vi "SocketQueue.vi"() -> (3 "SocketQueue":T1)   [LabVIEW 2018]
uses:
  SocketQueue.ctl
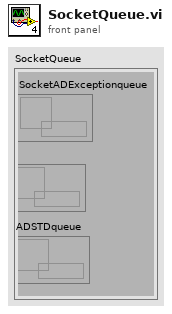
[diagram p1: front panel]
types:
  T1 = typedef "SocketQueue.ctl" = cluster{"ADSTDqueue ":refnum<queue>, "SocketADExceptionqueue":refnum<queue>, "  SocketAD":refnum<queue>}
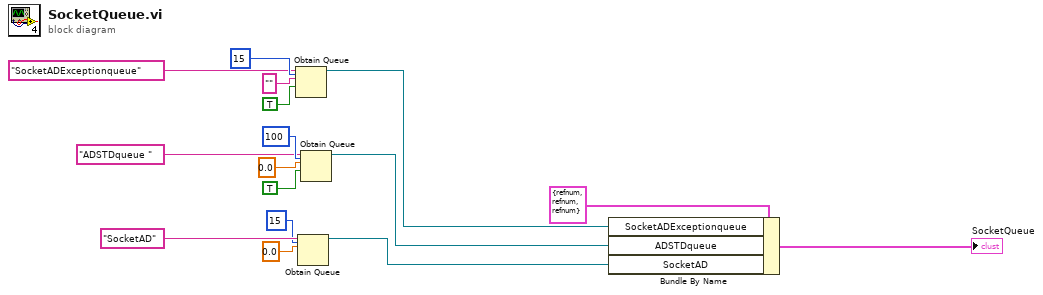
[diagram p0: block diagram]
diagram:
  n1 = Obtain Queue(max queue size (-1, unlimited)=15 ("队列最大值（-1，无限）"), name (unnamed)="SocketADExceptionqueue" ("名称（未命名）"), element data type="", create if not found? (T)=TRUE ("如未找到则创建？(T)")) -> (queue out=w8:refnum<queue>)  [unwired: 1 in, 2 out]
  n2 = Obtain Queue(max queue size (-1, unlimited)=15 ("队列最大值（-1，无限）"), name (unnamed)="SocketAD" ("名称（未命名）"), element data type=0.0) -> (queue out=w16:refnum<queue>)  [unwired: 2 in, 2 out]
  n3 = Obtain Queue(max queue size (-1, unlimited)=100 ("中值标准差队列长度"), name (unnamed)="ADSTDqueue " ("名称（未命名）"), element data type=0.0, create if not found? (T)=TRUE ("如未找到则创建？(T)")) -> (queue out=w12:refnum<queue>)  [unwired: 1 in, 2 out]
  n4 = Bundle By Name(cluster=T1 {"ADSTDqueue "=refnum, "SocketADExceptionqueue"=refnum, "  SocketAD"=refnum} ("簇"), "SocketADExceptionqueue"=w8, "ADSTDqueue"=w12, "SocketAD"=w16) -> (→"SocketQueue":T1)
